vi "KE6221 -- Wave Gen Example.vi"() -> ()   [LabVIEW 2020, in "Keithley 622x.lvlib"]
doc: "Example VI that shows how to set up and playback waveforms via a 6221."
uses:
  Keithley 622x.lvlib
  Utility/Typedefs/KE622x -- Instrument Type.ctl
  Configure/6221 Wave/Low Level/Typedefs/KE6221 -- Wave Type.ctl
  Configure/6221 Wave/Low Level/Typedefs/KE6221 -- Wave Frequency.ctl
  Configure/6221 Wave/Low Level/Typedefs/KE6221 -- Wave Amplitude.ctl
  Configure/6221 Wave/Low Level/Typedefs/KE6221 -- Wave Ranging Mode.ctl
  Configure/Source/Typedefs/KE622x -- Current Ranges.ctl
  Configure/6221 Wave/Low Level/Typedefs/KE6221 -- Wave Phase Marker.ctl
  C/Program Files/National Instruments/LabVIEW 2021/instr.lib/Keithley 622x LV 2009/Configure/Trigger/Low Level/Typedefs/KE622x -- Trig Link Line.ctl
  Configure/6221 Wave/Low Level/Typedefs/KE6221 -- Wave Playback Mode.ctl
  Configure/6221 Wave/Low Level/Typedefs/KE6221 -- Wave Playback Time.ctl
  Configure/6221 Wave/Low Level/Typedefs/KE6221 -- Wave Playback Num Cycles.ctl
  Configure/Source/Typedefs/KE622x -- Current Level.ctl
  C/Program Files/National Instruments/LabVIEW 2021/instr.lib/Keithley 622x LV 2009/Configure/6221 Wave/Typedefs/KE6221 -- Wave Sine Wave Params.ctl
  C/Program Files/National Instruments/LabVIEW 2021/instr.lib/Keithley 622x LV 2009/Configure/6221 Wave/Typedefs/KE6221 -- Wave Square Or Ramp Wave Select.ctl
  C/Program Files/National Instruments/LabVIEW 2021/instr.lib/Keithley 622x LV 2009/Configure/6221 Wave/Low Level/Typedefs/KE6221 -- Wave Duty Cycle.ctl
  C/Program Files/National Instruments/LabVIEW 2021/instr.lib/Keithley 622x LV 2009/Configure/6221 Wave/Typedefs/KE6221 -- Wave Square Or Ramp Wave Params.ctl
  Configure/6221 Wave/Low Level/Typedefs/KE6221 -- Arb Location.ctl
  Configure/6221 Wave/Low Level/Typedefs/KE6221 -- Wave Arb Point.ctl
  Configure/6221 Wave/Typedefs/KE6221 -- Wave Arb Wave Params.ctl
  C/Program Files/National Instruments/LabVIEW 2021/instr.lib/Keithley 622x LV 2009/Configure/6221 Wave/Typedefs/KE6221 -- Wave External Trig Params.ctl
  C/Program Files/National Instruments/LabVIEW 2021/instr.lib/Keithley 622x LV 2009/Configure/6221 Wave/Low Level/Typedefs/KE6221 -- Wave Extern Trig Link In Line.ctl
  C/Program Files/National Instruments/LabVIEW 2021/instr.lib/Keithley 622x LV 2009/Configure/6221 Wave/Low Level/Typedefs/KE6221 -- Wave Inactive Level.ctl
panel:
  out "Playback Completed Normally?":bool
  out "error out":errorcluster
  out "Waiting For Arm Layer Trig?":bool
  out "Waiting For Trig Layer Trig?":bool
  out "Playback Timeout?":bool
  out "Wave Mode Stopped?":bool
  out "Wave Mode Started?":bool
  in  "Playback Timeout (msecs)":u32=20000
  in  "External Trig Params":T1={"Ext Trig Enabled?"=FALSE, "Trig Link In Line"=enum."None", "Inactive Level (%)"=50.0, "Ignore Retrigs?"=FALSE} {"Inactive Level (%)" min=-100.0 max=100.0 format="%.3p"}
  in  "Tab Control":T4(tab)
  in  "Sine Wave Params":T5={"Frequency (Hz)"=1000.0, "Amplitude (A)"=0.001, "Offset (A)"=0.0, "Ranging Mode"=enum."Best", "Fixed Range"=enum."2mA", "Playback Mode"=enum."Num Cycles", "Time (s)"=1.0, "Num Cycles"=1.0, "Phase\nMarker?"=FALSE, "Phase Marker (deg)"=180.0, "Trig Link Line"=enum."1"} {"Offset (A)" min=-0.105 max=0.105 format="%.4p"; "Num Cycles" min=0.001 max=99999999900.0 format="%.3p"; "Time (s)" min=1e-07 max=999999.999 format="%.3p"; "Phase Marker (deg)" min=0.0 max=360.0 format="%.3f"; "Amplitude (A)" min=2e-12 max=0.105 format="%.3p"; "Frequency (Hz)" min=0.001 max=100000.0 format="%.3p"}
  in  "Square Or Ramp Wave Params In":T16={"Frequency (Hz)"=1000.0, "Amplitude (A)"=0.001, "Offset (A)"=0.0, "Duty Cycle (%)"=50.0, "Ranging Mode"=enum."Best", "Fixed Range"=enum."2mA", "Playback Mode"=enum."Time", "Time (s)"=1.0, "Num Cycles"=1.0, "Phase\nMarker?"=FALSE, "Phase Marker (deg)"=180.0, "Trig Link Line"=enum."1"} {"Duty Cycle (%)" min=0.0 max=100.0 format="%.3p"; "Offset (A)" min=-0.105 max=0.105 format="%.4p"; "Num Cycles" min=0.001 max=99999999900.0 format="%.3p"; "Time (s)" min=1e-07 max=999999.999 format="%.3p"; "Phase Marker (deg)" min=0.0 max=360.0 format="%.3f"; "Amplitude (A)" min=2e-12 max=0.105 format="%.3p"; "Frequency (Hz)" min=0.001 max=100000.0 format="%.3p"}
  in  "Square Wave Type":T18
  in  "Arb Wave Params In":T19={"Frequency (Hz)"=1000.0, "Amplitude (A)"=0.001, "Offset (A)"=0.0, "Ranging Mode"=enum."Best", "Fixed Range"=enum."2mA", "Playback Mode"=enum."Time", "Time (s)"=1.0, "Num Cycles"=1.0, "Phase\nMarker?"=FALSE, "Phase Marker (deg)"=180.0, "Trig Link Line"=enum."1", "Arb Waveform Points"=[], "Num Arb Points"=0} {"Arb Waveform Points" min=-1.0 max=1.0 format="%.3f"; "Offset (A)" min=-0.105 max=0.105 format="%.4p"; "Num Cycles" min=0.001 max=99999999900.0 format="%.3p"; "Time (s)" min=1e-07 max=999999.999 format="%.3p"; "Phase Marker (deg)" min=0.0 max=360.0 format="%.3f"; "Amplitude (A)" min=2e-12 max=0.105 format="%.3p"; "Frequency (Hz)" min=0.001 max=100000.0 format="%.3p"}
  in  "Arb Location":T21
  in  "Arb Waveform Load Timeout":u32=10000
  in  "Waveform Type":T22(ring)
  in  "Check For SCPI Errors? (T)":bool=TRUE
  in  "KE6221 Resource":refnum<visa-resource-name>
  # "Input"
  # "Output"
  # "Note:  \"Arb Waveform Points\" and \"Num Arb Points\" refer to the Arb waveform in volatile memory (a.k.a. 'Location 0'). For the 'set' VI, the points are automatically copied into the specified non-volatile memory location."
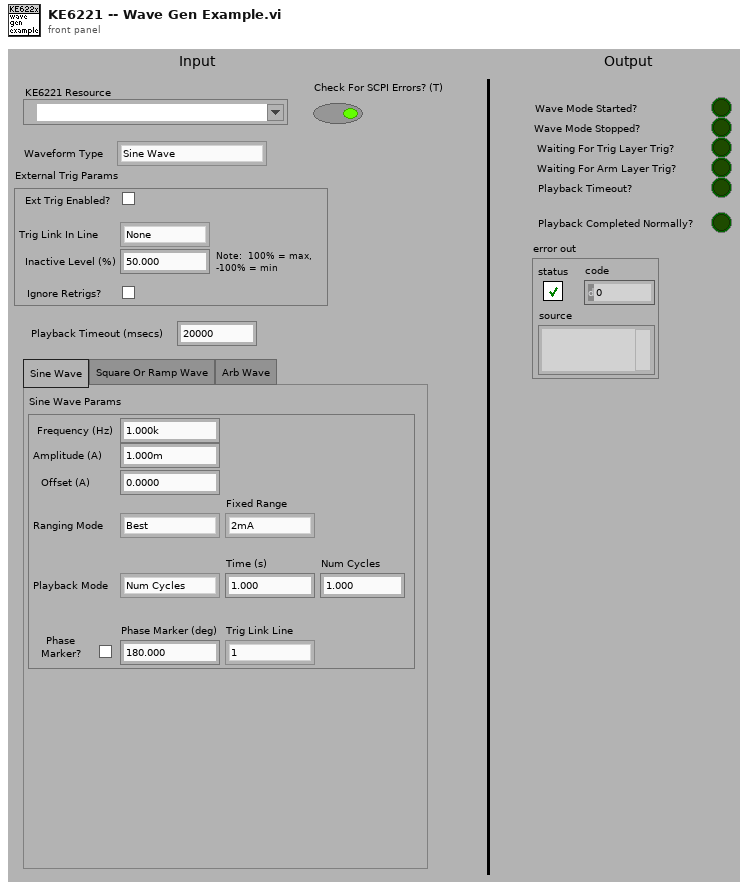
[diagram p1: front panel]
types:
  T1 = typedef "Keithley 622x.lvlib/KE6221 -- Wave External Trig Params.ctl" = cluster{"Ext Trig Enabled?":bool, "Trig Link In Line":T2, "Inactive Level (%)":T3, "Ignore Retrigs?":bool}
  T2 = typedef "Keithley 622x.lvlib/KE6221 -- Wave Extern Trig Link In Line.ctl" = enum16{"None", "1", "2", "3", "4", "5", "6"}
  T3 = typedef "Keithley 622x.lvlib/KE6221 -- Wave Inactive Level.ctl" = dbl
  T4 = enum32{"Sine Wave", "Square Or Ramp Wave", "Arb Wave"}
  T5 = typedef "Keithley 622x.lvlib/KE6221 -- Wave Sine Wave Params.ctl" = cluster{"Frequency (Hz)":T6, "Amplitude (A)":T7, "Offset (A)":T8, "Ranging Mode":T9, "Fixed Range":T10, "Playback Mode":T11, "Time (s)":T12, "Num Cycles":T13, "Phase\nMarker?":bool, "Phase Marker (deg)":T14, "Trig Link Line":T15}
  T6 = typedef "Keithley 622x.lvlib/KE6221 -- Wave Frequency.ctl" = dbl
  T7 = typedef "Keithley 622x.lvlib/KE6221 -- Wave Amplitude.ctl" = dbl
  T8 = typedef "Keithley 622x.lvlib/KE622x -- Current Level.ctl" = dbl
  T9 = typedef "Keithley 622x.lvlib/KE6221 -- Wave Ranging Mode.ctl" = enum16{"Best", "Fixed"}
  T10 = typedef "Keithley 622x.lvlib/KE622x -- Current Ranges.ctl" = enum16{"2nA", "20nA", "200nA", "2uA", "20uA", "200uA", "2mA", "20mA", "100mA"}
  T11 = typedef "Keithley 622x.lvlib/KE6221 -- Wave Playback Mode.ctl" = enum16{"Time", "Num Cycles"}
  T12 = typedef "Keithley 622x.lvlib/KE6221 -- Wave Playback Time.ctl" = dbl
  T13 = typedef "Keithley 622x.lvlib/KE6221 -- Wave Playback Num Cycles.ctl" = dbl
  T14 = typedef "Keithley 622x.lvlib/KE6221 -- Wave Phase Marker.ctl" = dbl
  T15 = typedef "Keithley 622x.lvlib/KE622x -- Trig Link Line.ctl" = enum16{"1", "2", "3", "4", "5", "6"}
  T16 = typedef "Keithley 622x.lvlib/KE6221 -- Wave Square Or Ramp Wave Params.ctl" = cluster{"Frequency (Hz)":T6, "Amplitude (A)":T7, "Offset (A)":T8, "Duty Cycle (%)":T17, "Ranging Mode":T9, "Fixed Range":T10, "Playback Mode":T11, "Time (s)":T12, "Num Cycles":T13, "Phase\nMarker?":bool, "Phase Marker (deg)":T14, "Trig Link Line":T15}
  T17 = typedef "Keithley 622x.lvlib/KE6221 -- Wave Duty Cycle.ctl" = dbl
  T18 = typedef "Keithley 622x.lvlib/KE6221 -- Wave Square Or Ramp Wave Select.ctl" = enum16{"Square", "Ramp"}
  T19 = typedef "Keithley 622x.lvlib/KE6221 -- Wave Arb Wave Params.ctl" = cluster{"Frequency (Hz)":T6, "Amplitude (A)":T7, "Offset (A)":T8, "Ranging Mode":T9, "Fixed Range":T10, "Playback Mode":T11, "Time (s)":T12, "Num Cycles":T13, "Phase\nMarker?":bool, "Phase Marker (deg)":T14, "Trig Link Line":T15, "Arb Waveform Points":T20[], "Num Arb Points":u32}
  T20 = typedef "Keithley 622x.lvlib/KE6221 -- Wave Arb Point.ctl" = dbl
  T21 = typedef "Keithley 622x.lvlib/KE6221 -- Arb Location.ctl" = enum16{"0 (Volatile)", "1 (NVRAM)", "2 (NVRAM)", "3 (NVRAM)", "4 (NVRAM)"}
  T22 = enum16{"Sine Wave", "Square Or Ramp Wave", "Arb Wave"}
  T23 = typedef "Keithley 622x.lvlib/KE622x -- Instrument Type.ctl" = enum16{"KE6220", "KE6221"}
  T24 = typedef "Keithley 622x.lvlib/KE6221 -- Wave Type.ctl" = enum16{"Sinusoid", "Square", "Ramp", "Arbitrary 0", "Arbitrary 1", "Arbitrary 2", "Arbitrary 3", "Arbitrary 4"}
  T25 = typedef "Keithley 622x.lvlib/KE622x -- Op Event Reg State.ctl" = cluster{"B0, CAL:  Instrument Calibrating Event?":bool, "B1, SwpD:  Sweep, Delta, Diff Cond, or Pulse Sweep Complete Event?":bool, "B2, SwpA:  Sweep, Delta, Diff Cond, or Pulse Sweep Aborted Event?":bool, "B3, Swp:  Sweep, Delta, Diff Cond, or Pulse Sweep Sweeping Event?":bool, "B4, WStrt:  KE6221 Wave Mode Started Event?":bool, "B5, Trig:  Waiting For Trigger Event Event?":bool, "B6, Arm:  Waiting For Arm Event Event?":bool, "B7, Wstop:  KE6221 Wave Mode Aborted Event?":bool, "B8, Filt:  Delta Test Started And Filter Settled Event?":bool, "B10, Idle:  Idle State Event?":bool, "B11, RSE:  RS-232 Error Event?":bool}
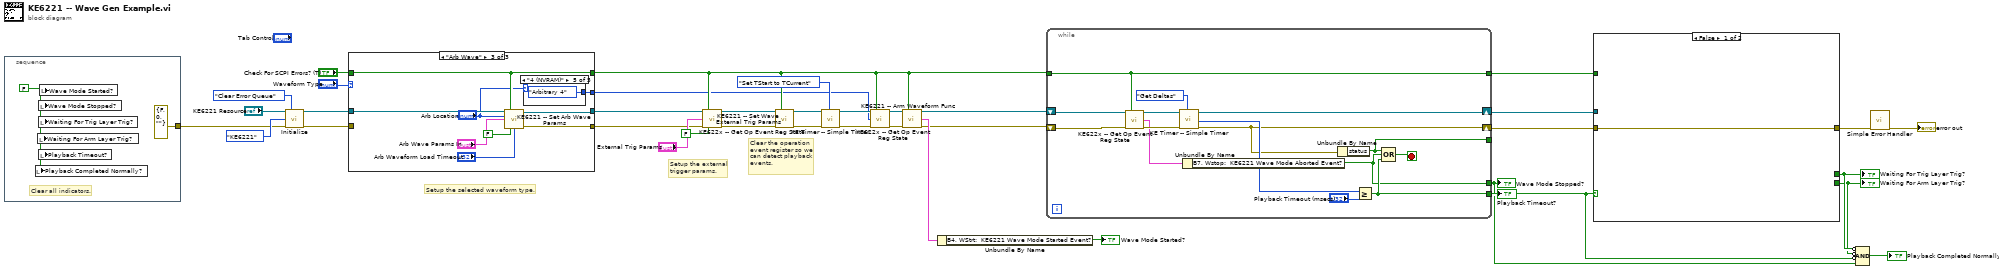
[diagram p0: block diagram]
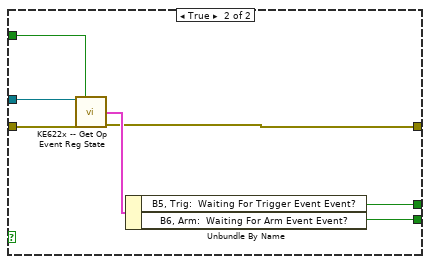
[diagram p2: hidden frame]
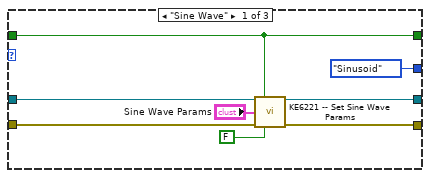
[diagram p3: hidden frame]
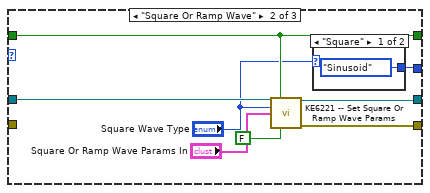
[diagram p4: hidden frame]
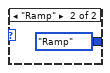
[diagram p5: hidden frame]
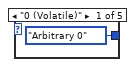
[diagram p6: hidden frame]
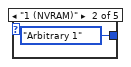
[diagram p7: hidden frame]
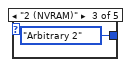
[diagram p8: hidden frame]
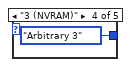
[diagram p9: hidden frame]
diagram:
  # "Clear the operation\nevent register so we\ncan detect playback\nevents."
  # "Setup the external\ntrigger params."
  # "Setup the selected waveform type."
  n1 = stacked-sequence {
    tunnel: [errorcluster {"status"=FALSE, "code"=0, "source"=""} ("error in (no error)")] -> w1
    frame #0 {
      w39 = FALSE
      # "Clear all indicators."
      n2 = local write "Playback Completed Normally?"(w39) -> ()
      n3 = local write "Waiting For Arm Layer Trig?"(w39) -> ()
      n4 = local write "Wave Mode Stopped?"(w39) -> ()
      n5 = local write "Waiting For Trig Layer Trig?"(w39) -> ()
      n6 = local write "Playback Timeout?"(w39) -> ()
      n7 = local write "Wave Mode Started?"(w39) -> ()
    }
  }
  n8 = call "Initialize.vi"("VISA resource name"="KE6221 Resource", "Error Queue Option"=enum16{"Clear Error Queue", "Error Query"}."Clear Error Queue", "Instrument Type"=KE622x_--_Instrument_Type."KE6221", "error in (no error)"=w1) -> ("VISA resource name out"=w31:refnum<visa-resource-name>, "error out"=w28:errorcluster)  [unwired: 10 in]
  n9 = case shown="\"Arb Wave\"" "Waveform Type" {
    tunnel: w31 -> [w47 w55 w66]
    tunnel: "Check For SCPI Errors? (T)" -> [w42 w50 w60]
    tunnel: [w44 w53 w65] -> w34
    tunnel: [w43 w52 w64] -> w33
    tunnel: [w42 w50 w60] -> w17
    tunnel: w28 -> [w41 _ _]
    tunnel: [KE6221_--_Wave_Type."Sinusoid" ("Wave Type") w48 w58] -> w7
    frame "Sine Wave" {
      n10 = call "KE6221 -- Set Sine Wave Params.vi"("Resource In"=w47, "Check For SCPI Errors? (T)"=w42, "Sine Wave Params In"="Sine Wave Params", "error in (no error)"=w41, "Read Back Set Values? (T)"=FALSE) -> ("Resource Out (dupl)"=w44:refnum<visa-resource-name>, "error out"=w43:errorcluster)  [unwired: 8 in, 1 out]
    }
    frame "Square Or Ramp Wave" {
      n11 = call "KE6221 -- Set Square Or Ramp Wave Params.vi"("Resource In"=w55, "Check For SCPI Errors? (T)"=w50, "Wave Type In"="Square Wave Type", "Square Or Ramp Wave Params In"="Square Or Ramp Wave Params In", "Read Back Set Values? (T)"=FALSE) -> ("Resource Out (dupl)"=w53:refnum<visa-resource-name>, "error out"=w52:errorcluster)  [unwired: 8 in, 1 out]
      n12 = case shown="\"Square\"" "Square Wave Type" {
        tunnel: [KE6221_--_Wave_Type."Sinusoid" ("Wave Type") KE6221_--_Wave_Type."Ramp" ("Wave Type")] -> w48
        frame "Square" {
        }
        frame "Ramp" {
        }
      }
    }
    frame "Arb Wave" {
      n13 = call "KE6221 -- Set Arb Wave Params.vi"("Resource In"=w66, "Check For SCPI Errors? (T)"=w60, "Arb Location"="Arb Location", "Arb Wave Params In"="Arb Wave Params In", "Read Back Set Values? (T)"=FALSE, "Timeout (10000 ms)"="Arb Waveform Load Timeout") -> ("Resource Out (dupl)"=w65:refnum<visa-resource-name>, "error out"=w64:errorcluster)  [unwired: 7 in, 1 out]
      n14 = case shown="\"4 (NVRAM)\"" "Arb Location" {
        tunnel: [KE6221_--_Wave_Type."Arbitrary 0" ("Wave Type") KE6221_--_Wave_Type."Arbitrary 1" ("Wave Type") KE6221_--_Wave_Type."Arbitrary 2" ("Wave Type") KE6221_--_Wave_Type."Arbitrary 3" ("Wave Type") KE6221_--_Wave_Type."Arbitrary 4" ("Wave Type")] -> w58
        frame "0 (Volatile)" {
        }
        frame "1 (NVRAM)" {
        }
        frame "2 (NVRAM)" {
        }
        frame "3 (NVRAM)" {
        }
        frame "4 (NVRAM)" {
        }
      }
    }
  }
  n15 = call "KE6221 -- Set Wave External Trig Params.vi"("Resource In"=w34, "Check For SCPI Errors? (T)"=w17, "External Trig Params In"="External Trig Params", "error in (no error)"=w33, "Read Back Set Values? (T)"=FALSE) -> ("Resource Out (dupl)"=w27:refnum<visa-resource-name>, "error out"=w26:errorcluster)  [unwired: 8 in, 1 out]
  n16 = call "KE622x -- Get Op Event Reg State.vi"("VISA Resource In"=w27, "Error Query (T)?"=w17, "error in (no error)"=w26) -> ("VISA Resource Out (dupl)"=w22:refnum<visa-resource-name>, "error out"=w21:errorcluster)  [unwired: 10 in, 1 out]
  n17 = call "KE Timer -- Simple Timer.vi"("Resource In"=w22, "error in (no error)"=w21, "Action"=enum16{"Set TStart to TCurrent", "Get Deltas"}."Set TStart to TCurrent") -> ("Resource Out (dupl)"=w24:refnum<visa-resource-name>, "error out (dupl)"=w23:errorcluster)  [unwired: 7 in, 8 out]
  n18 = call "KE6221 -- Arm Waveform Func.vi"("Resource In"=w24, "Check For SCPI Errors? (T)"=w17, "Wave Type"=w7, "error in (no error)"=w23) -> ("Resource Out (dupl)"=w19:refnum<visa-resource-name>, "error out"=w18:errorcluster)  [unwired: 10 in]
  n19 = call "KE622x -- Get Op Event Reg State.vi"("VISA Resource In"=w19, "Error Query (T)?"=w17, "error in (no error)"=w18) -> ("VISA Resource Out (dupl)"=w14:refnum<visa-resource-name>, "KE622x Op Event Reg"=w16:T25, "error out"=w13:errorcluster)  [unwired: 10 in]
  n20 = Unbundle By Name(w16) -> ("B4, WStrt:  KE6221 Wave Mode Started Event?"=→"Wave Mode Started?":bool)
  n21 = while {
    shift-right: [w77] -> w11
    shift-left: w13 -> [w74]
    shift-right: [w78] -> w12
    shift-left: w14 -> [w75]
    tunnel: w17 -> [w73]
    tunnel: [w79] -> w4
    tunnel: [w76] -> _
    tunnel: [w73] -> w10
    tunnel: [w72] -> w3
    stop <- w80 stop-if-true
    n22 = call "KE622x -- Get Op Event Reg State.vi"("VISA Resource In"=w75, "Error Query (T)?"=w73, "error in (no error)"=w74) -> ("VISA Resource Out (dupl)"=w86:refnum<visa-resource-name>, "KE622x Op Event Reg"=w81:T25, "error out"=w85:errorcluster)  [unwired: 10 in]
    n23 = call "KE Timer -- Simple Timer.vi"("Resource In"=w86, "error in (no error)"=w85, "Action"=enum16{"Set TStart to TCurrent", "Get Deltas"}."Get Deltas") -> ("Resource Out (dupl)"=w78:refnum<visa-resource-name>, "TCurrent - TStart (ms)"=w83:u32, "error out (dupl)"=w77:errorcluster)  [unwired: 7 in, 7 out]
    n24 = Unbundle By Name(w81) -> ("B7, Wstop:  KE6221 Wave Mode Aborted Event?"=w72:bool)
    n25 = Unbundle By Name(w77) -> ("status"=w76:bool)
    n26 = Greater Or Equal?(x=w83, y="Playback Timeout (msecs)") -> (x >= y?=w79:bool)
    n27 = Compound Arithmetic op=OR(w76, w72, w79) -> (w80:bool)
  }
  "Wave Mode Stopped?" <- w3
  "Playback Timeout?" <- w4
  n28 = case shown="False" w4 {
    tunnel: w12 -> [_ w94]
    tunnel: w11 -> [w87 w93]
    tunnel: w10 -> [_ w88]
    tunnel: [_ w91] -> w6
    tunnel: [_ w90] -> w5
    tunnel: [w87 w89] -> w9
    frame False {
    }
    frame True {
      n29 = call "KE622x -- Get Op Event Reg State.vi"("VISA Resource In"=w94, "Error Query (T)?"=w88, "error in (no error)"=w93) -> ("KE622x Op Event Reg"=w92:T25, "error out"=w89:errorcluster)  [unwired: 10 in, 1 out]
      n30 = Unbundle By Name(w92) -> ("B5, Trig:  Waiting For Trigger Event Event?"=w91:bool, "B6, Arm:  Waiting For Arm Event Event?"=w90:bool)
    }
  }
  "Waiting For Trig Layer Trig?" <- w6
  "Waiting For Arm Layer Trig?" <- w5
  n31 = Compound Arithmetic op=AND(invert w6, invert w5, invert w4, w3) -> (→"Playback Completed Normally?":bool)
  n32 = call <vilib>:"Simple Error Handler.vi"("error in (no error)"=w9) -> ("error out"=→"error out":errorcluster)  [unwired: 4 in, 4 out]
